vi "matrix_vector_product (SubVI).vi"(6 "Input vector":sgl[](array[numeric]), 9 "Line 3":sgl[](array[numeric])=[0.0, 0.0, 0.0], 10 "Line 2":sgl[](array[numeric])=[0.0, 0.0, 0.0], 11 "Line 1":sgl[](array[numeric])=[0.0, 0.0, 0.0]) -> (3 "Output vector":sgl[](array[numeric]))   [LabVIEW 2011]
panel:
  # "Input Matrix"
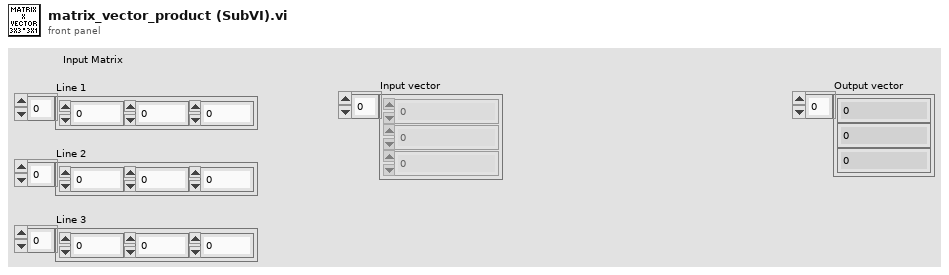
[diagram p1: front panel]
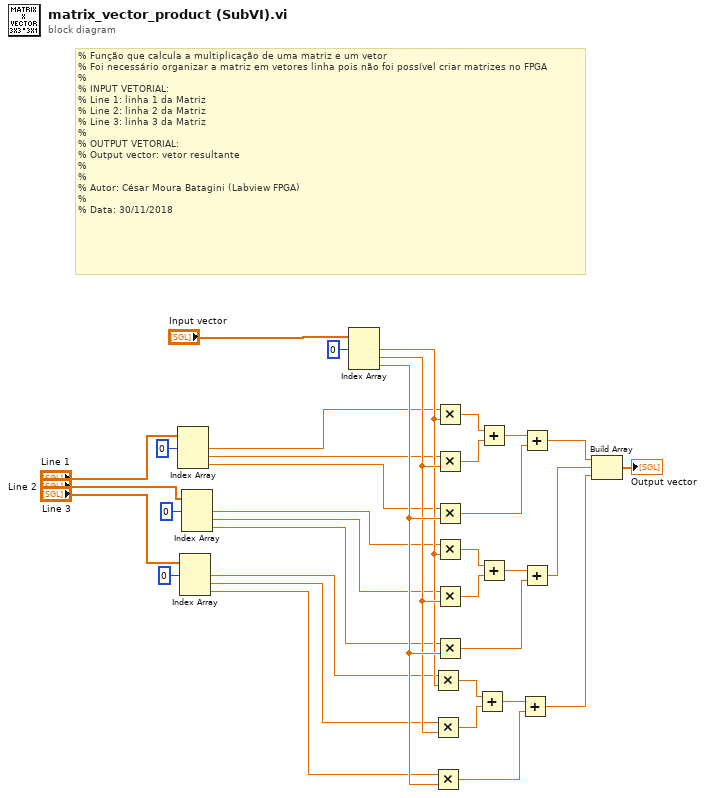
[diagram p0: block diagram]
diagram:
  # "% Função que calcula a multiplicação de uma matriz e um vetor\n% Foi necessário organizar a matriz em vetores linha pois não foi possível criar matrizes no FPGA\n%\n% INPUT VETORIAL: \n% Line 1: linha 1 da Matriz\n% Line 2: linha 2 da Matriz\n% Line 3: linha 3 da Matriz\n%\n% OUTPUT VETORIAL:\n% Output vector: vetor resultante\n%\n%\n% Autor: César Moura Batagini (Labview FPGA)\n%             \n% Data: 30/11/2018"
  n1 = Index Array(array="Line 1", index #1=0 ("index")) -> (element #1=w9:sgl, element #2=w10:sgl, element #3=w11:sgl)  [unwired: 2 in]
  n2 = Index Array(array="Line 3", index #1=0 ("index")) -> (element #1=w27:sgl, element #2=w28:sgl, element #3=w29:sgl)  [unwired: 2 in]
  n3 = Index Array(array="Line 2", index #1=0 ("index")) -> (element #1=w24:sgl, element #2=w25:sgl, element #3=w26:sgl)  [unwired: 2 in]
  n4 = Index Array(array="Input vector", index #1=0 ("index")) -> (element #1=w30:sgl, element #2=w31:sgl, element #3=w32:sgl)  [unwired: 2 in]
  n5 = Multiply(x=w27, y=w30) -> (x*y=w20:sgl)
  n6 = Multiply(x=w28, y=w31) -> (x*y=w21:sgl)
  n7 = Multiply(x=w29, y=w32) -> (x*y=w23:sgl)
  n8 = Multiply(x=w9, y=w30) -> (x*y=w12:sgl)
  n9 = Multiply(x=w10, y=w31) -> (x*y=w13:sgl)
  n10 = Multiply(x=w11, y=w32) -> (x*y=w15:sgl)
  n11 = Multiply(x=w24, y=w30) -> (x*y=w19:sgl)
  n12 = Multiply(x=w25, y=w31) -> (x*y=w18:sgl)
  n13 = Multiply(x=w26, y=w32) -> (x*y=w16:sgl)
  n14 = Add(x=w20, y=w21) -> (x+y=w22:sgl)
  n15 = Add(x=w12, y=w13) -> (x+y=w14:sgl)
  n16 = Add(x=w19, y=w18) -> (x+y=w17:sgl)
  n17 = Add(x=w22, y=w23) -> (x+y=w35:sgl)
  n18 = Add(x=w14, y=w15) -> (x+y=w33:sgl)
  n19 = Add(x=w17, y=w16) -> (x+y=w34:sgl)
  n20 = Build Array(w33, w34, w35) -> (→"Output vector":sgl[])
